vi "test_calc-edeg_omega.vi"() -> ()   [LabVIEW 2019]
uses:
  <vilib>/Analysis/Matrix/Datatypes/RealMatrix.ctl
  <vilib>/Analysis/coordinate.llb/Euler Rotation Order.ctl
  <vilib>/Analysis/Matrix/Numeric/Conversions/Array To Matrix - RA2.vi
  <vilib>/Analysis/Matrix/Numeric/Multiply/Multiply - RM,RM.vi
  <vilib>/Analysis/Matrix/Numeric/Add/Add - RM,RM.vi
  <vilib>/Analysis/baseanly.llb/Real Inverse Matrix.vi
  <vilib>/Analysis/NI_AALPro.lvlib
  <vilib>/Analysis/Matrix/NI_Matrix.lvlib
  <vilib>/Analysis/NI_AALBase.lvlib
panel:
  out "A * B":T1 caption="check11"
  out "check2":T1 caption="A * B"
  out "check1":T1 caption="A * B"
  out "edge.omega":T1=[[49.99999999999999, -1.3007944362217067e-15, 0.0], [1.2180969111322443e-15, 49.99999999999999, 0.0], [-0.0, -0.0, 1641.403175005872]] caption="역행렬"
  in  "tangle 2":dbl=-0.5953987473168079 format="%#_13g"
  in  "tangle 1":dbl=-0.44510127361856844 format="%#_13g"
  out "Rt2":T1=[[0.8279249316460434, 0.5608389319215406, 0.0], [-0.5608389319215406, 0.8279249316460434, 0.0], [0.0, 0.0, 1.0]] caption="rt2"
  out "Real Rt1":T1=[[0.9025670667402838, 0.43054928874153325, 0.0], [-0.43054928874153325, 0.9025670667402838, 0.0], [0.0, 0.0, 1.0]] caption="rt1"
  out "sigma":T1=[[0.010000000000000002, 0.0, 0.0], [0.0, 0.010000000000000002, 0.0], [0.0, 0.0, 0.00030461741978670857]]
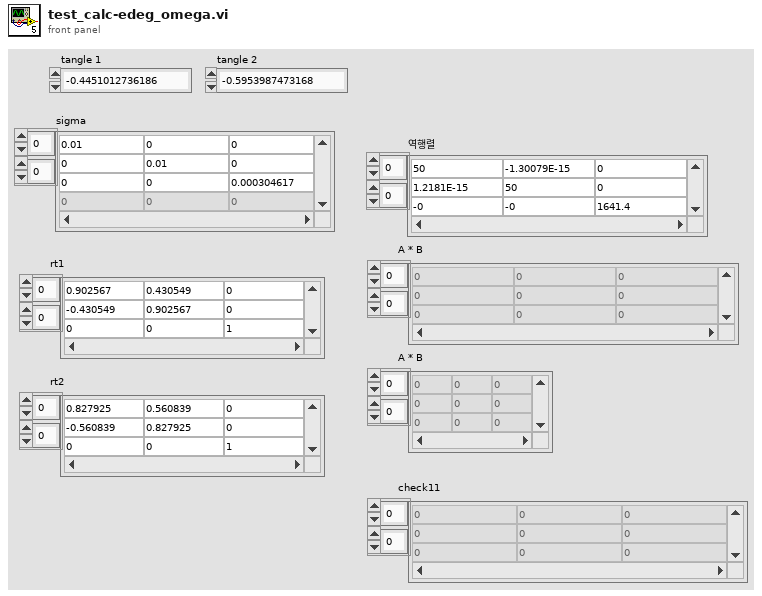
[diagram p1: front panel]
types:
  T1 = typedef "NI_Matrix.lvlib/RealMatrix.ctl" = dbl[][]
  T2 = typedef "NI_AALPro.lvlib/Euler Rotation Order.ctl" = u16
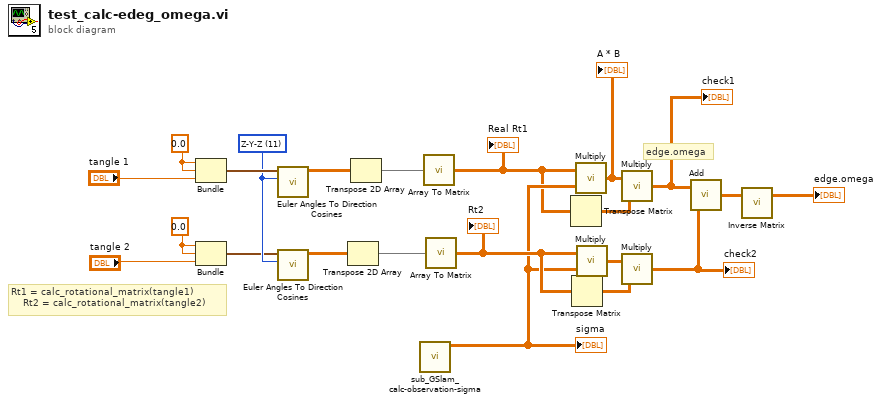
[diagram p0: block diagram]
diagram:
  w19 = T2 11 items=["X-Y-Z", "X-Z-Y", "Y-X-Z", "Y-Z-X", "Z-X-Y", "Z-Y-X", "X-Y-X", "X-Z-X", "Y-X-Y", "Y-Z-Y", "Z-X-Z", "Z-Y-Z"] ("rotation order")
  w21 = 0.0 ("원소")
  w22 = 0.0 ("원소")
  # "edge.omega"
  # "Rt1 = calc_rotational_matrix(tangle1)\n    Rt2 = calc_rotational_matrix(tangle2)"
  n1 = Bundle("원소"=w22, "원소"=w22, "tangle 1"="tangle 1") -> (w20:cluster{"원소":dbl, "원소":dbl, "tangle 1":dbl})  [unwired: 1 in]
  n2 = Bundle("원소"=w21, "원소"=w21, "tangle 2"="tangle 2") -> (w18:cluster{"원소":dbl, "원소":dbl, "tangle 2":dbl})  [unwired: 1 in]
  n3 = call <vilib>:"Euler Angles To Direction Cosines.vi"("rotation order"=w19, "Euler Angles"=w20) -> ("Direction Cosines"=w17:dbl[][])  [unwired: 8 in, 1 out]
  n4 = call <vilib>:"Euler Angles To Direction Cosines.vi"("rotation order"=w19, "Euler Angles"=w18) -> ("Direction Cosines"=w13:dbl[][])  [unwired: 8 in, 1 out]
  n5 = Transpose 2D Array(2D array=w13) -> (transposed array=w7:dbl[][])
  n6 = Transpose 2D Array(2D array=w17) -> (transposed array=w8:dbl[][])
  n7 = call "sub_GSlam_calc-observation-sigma.vi"() -> ("sigma"=w3:T1)  [unwired: 11 in]
  "sigma" <- w3
  n8 = call-poly <vilib>:"Array To Matrix.vi"("Real 2D Array"=w8) -> ("Real Matrix"=w1:T1)
  "Real Rt1" <- w1
  n9 = call-poly <vilib>:"Array To Matrix.vi"("Real 2D Array"=w7) -> ("Real Matrix"=w12:T1)
  "Rt2" <- w12
  n10 = Transpose Matrix(1:w1) -> (0:w2:T1)
  n11 = Transpose Matrix(1:w12) -> (0:w15:T1)
  n12 = call-poly <vilib>:"Multiply.vi"("Real Matrix B"=w3, "Real Matrix A"=w1) -> ("A * B"=w16:T1)
  "A * B" <- w16
  n13 = call-poly <vilib>:"Multiply.vi"("Real Matrix B"=w3, "Real Matrix A"=w12) -> ("A * B"=w14:T1)
  n14 = call-poly <vilib>:"Multiply.vi"("Real Matrix B"=w2, "Real Matrix A"=w16) -> ("A * B"=w11:T1)
  "check1" <- w11
  n15 = call-poly <vilib>:"Multiply.vi"("Real Matrix B"=w15, "Real Matrix A"=w14) -> ("A * B"=w10:T1)
  "check2" <- w10
  n16 = call-poly <vilib>:"Add.vi"("Real Matrix B"=w10, "Real Matrix A"=w11) -> ("A + B"=w9:T1)
  n17 = call-poly <vilib>:"Inverse Matrix.vi"("Input Matrix"=w9) -> ("Inverse Matrix"=→"edge.omega":T1)  [unwired: 1 in, 1 out]
